vi "Message Parser Main.vi"(8 "error in (no error)":errorcluster, 11 "Message":T1={"Payload Size"=0, "Sequence Number"=0, "Sensor Type"=enum."APP", "Message Types"=enum."SEND_LOG_FILE_SIZE", "Data"=[]}) -> (0 "error out":errorcluster)   [LabVIEW 2019]
uses:
  Typedefs/Message.ctl
  Typedefs/Sensor Types.ctl
  Typedefs/Message Types.ctl
  Comms/State Controller/Controls/Comms Loop States.ctl
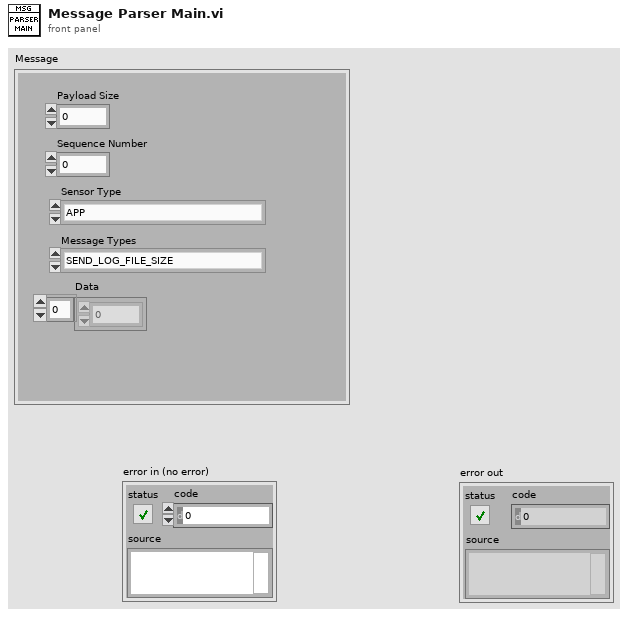
[diagram p1: front panel]
types:
  T1 = typedef "Message.ctl" = cluster{"Payload Size":u8, "Sequence Number":u8, "Sensor Type":T2, "Message Types":T3, "Data":u8[]}
  T2 = typedef "Sensor Types.ctl" = enum16{"APP", "TURBIDITY", "PH"}
  T3 = typedef "Message Types.ctl" = enum16{"HEART_BEAT", "CONNECT", "GET_CURRENT_MEASUREMENTS", "GET_LOG_FILE", "SEND_LOG_FILE_SIZE", "SEND_LOG_FILE_CHUNK", "GET_LOGGING_PERIOD", "SET_LOGGING_PERIOD", "SEND_SD_CARD_INFO", "GET_LOGS_LIST", "SEND_LOG_FILE_NAME", "SEND_LOGGING_PERIOD", "GET_RTC_TIME", "SET_RTC_TIME", "SEND_RTC_TIME", "SEND_CURRENT_MEASUREMENTS", "DELETE_LOG_FILE", "GET_SD_CARD_INFO", "GET_BATTERY_INFO", "SEND_BATTERY_INFO", "GET_LOG_FILE_SIZE", "SET_WIFI_SSID", "SET_WIFI_PASSWORD", "GET_WIFI_DETAILS", "SEND_WIFI_DETAILS", "ERROR_MSG"}
  T4 = typedef "Comms Loop States.ctl" = enum16{"Initalise", "User Event", "HEART_BEAT", "SEND_LOG_FILE_NAME", "Clear Log File Names", "SEND_LOG_FILE_CHUNK", "SEND_LOG_FILE_SIZE", "SEND_SD_CARD_INFO", "SEND_BATTERY_INFO", "SEND_LOGGING_PERIOD", "SEND_RTC_TIME", "SEND_CURRENT_MEASUREMENTS", "ERROR_MSG", "Clear Error Messages", "Send Message", "Idle", "Sensor Connected", "Sensor Disconnected", "Set Page Displayed", "Set Connected Sensor Type", "UI: Update Sensor Type", "UI: Update Log List", "Reset Log File Transfer", "SEND_WIFI_DETAILS"}
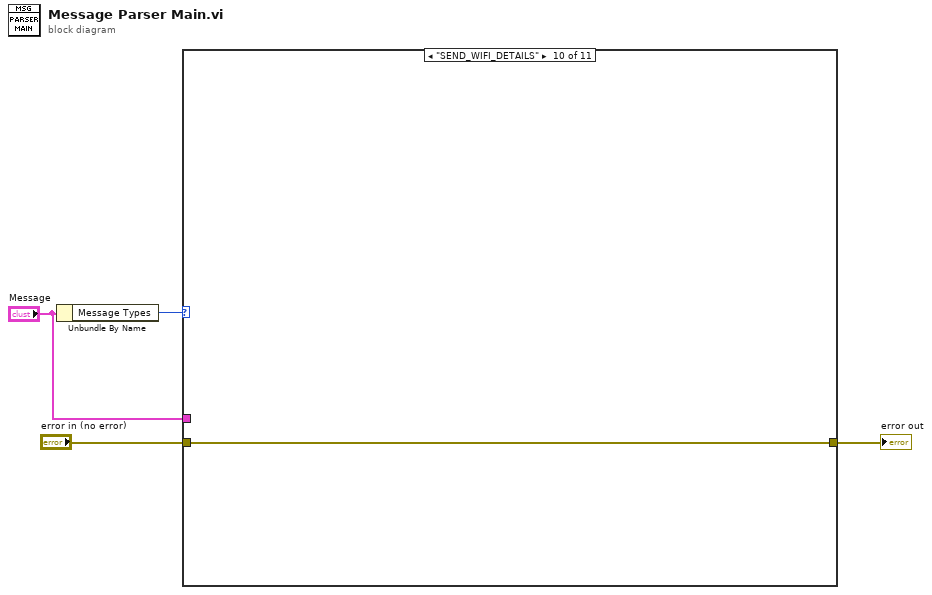
[diagram p0: block diagram]
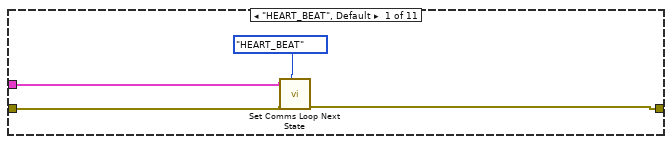
[diagram p2: hidden frame]
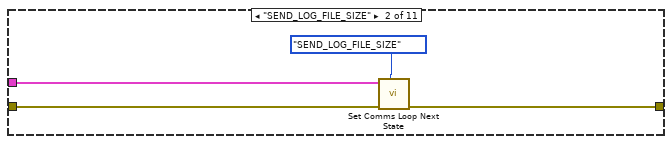
[diagram p3: hidden frame]
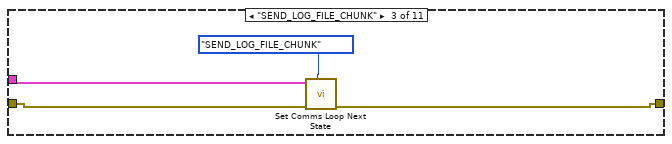
[diagram p4: hidden frame]
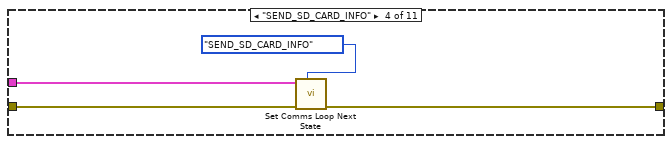
[diagram p5: hidden frame]
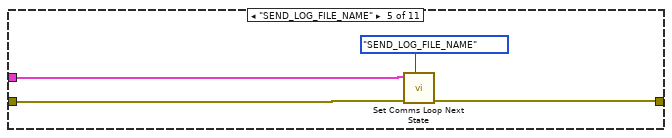
[diagram p6: hidden frame]
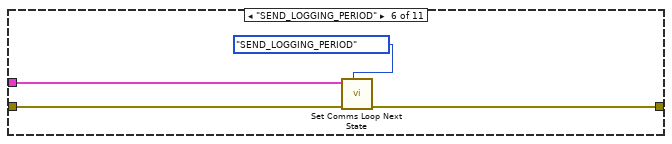
[diagram p7: hidden frame]
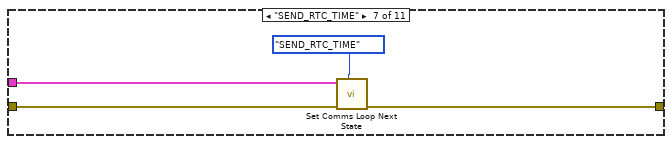
[diagram p8: hidden frame]
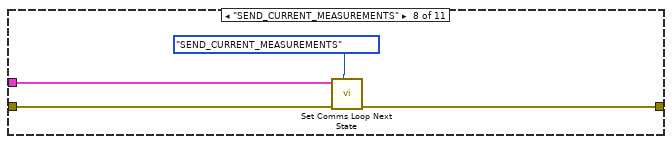
[diagram p9: hidden frame]
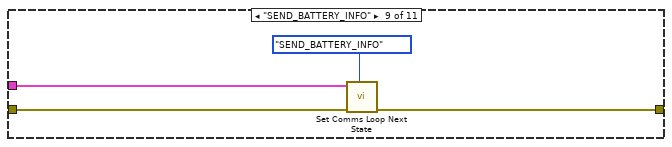
[diagram p10: hidden frame]
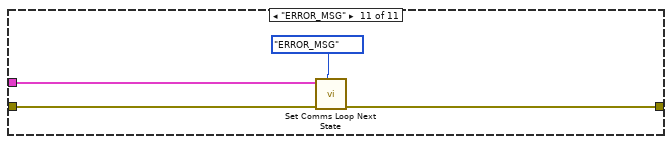
[diagram p11: hidden frame]
diagram:
  n1 = Unbundle By Name("Message") -> ("Message Types"=w2:T3)
  n2 = case shown="\"SEND_WIFI_DETAILS\"" w2 {
    tunnel: [w5 w9 w13 w17 w23 w25 w29 w34 w37 w41 w42] -> w4
    tunnel: "error in (no error)" -> [w7 w10 w15 w18 w22 w27 w31 w35 w39 w41 w44]
    tunnel: "Message" -> [w6 w11 w14 w19 w21 w26 w30 w33 w38 _ w43]
    frame "HEART_BEAT", Default {
      n3 = call "Set Comms Loop Next State.vi"("Command"=Comms_Loop_States."HEART_BEAT", "error in (no error)"=w7, "Data"=w6) -> ("error out"=w5:errorcluster)  [unwired: 8 in]
    }
    frame "SEND_LOG_FILE_SIZE" {
      n4 = call "Set Comms Loop Next State.vi"("Command"=Comms_Loop_States."SEND_LOG_FILE_SIZE", "error in (no error)"=w10, "Data"=w11) -> ("error out"=w9:errorcluster)  [unwired: 8 in]
    }
    frame "SEND_LOG_FILE_CHUNK" {
      n5 = call "Set Comms Loop Next State.vi"("Command"=Comms_Loop_States."SEND_LOG_FILE_CHUNK", "error in (no error)"=w15, "Data"=w14) -> ("error out"=w13:errorcluster)  [unwired: 8 in]
    }
    frame "SEND_SD_CARD_INFO" {
      n6 = call "Set Comms Loop Next State.vi"("Command"=Comms_Loop_States."SEND_SD_CARD_INFO", "error in (no error)"=w18, "Data"=w19) -> ("error out"=w17:errorcluster)  [unwired: 8 in]
    }
    frame "SEND_LOG_FILE_NAME" {
      n7 = call "Set Comms Loop Next State.vi"("Command"=Comms_Loop_States."SEND_LOG_FILE_NAME", "error in (no error)"=w22, "Data"=w21) -> ("error out"=w23:errorcluster)  [unwired: 8 in]
    }
    frame "SEND_LOGGING_PERIOD" {
      n8 = call "Set Comms Loop Next State.vi"("Command"=Comms_Loop_States."SEND_LOGGING_PERIOD", "error in (no error)"=w27, "Data"=w26) -> ("error out"=w25:errorcluster)  [unwired: 8 in]
    }
    frame "SEND_RTC_TIME" {
      n9 = call "Set Comms Loop Next State.vi"("Command"=Comms_Loop_States."SEND_RTC_TIME", "error in (no error)"=w31, "Data"=w30) -> ("error out"=w29:errorcluster)  [unwired: 8 in]
    }
    frame "SEND_CURRENT_MEASUREMENTS" {
      n10 = call "Set Comms Loop Next State.vi"("Command"=Comms_Loop_States."SEND_CURRENT_MEASUREMENTS", "error in (no error)"=w35, "Data"=w33) -> ("error out"=w34:errorcluster)  [unwired: 8 in]
    }
    frame "SEND_BATTERY_INFO" {
      n11 = call "Set Comms Loop Next State.vi"("Command"=Comms_Loop_States."SEND_BATTERY_INFO", "error in (no error)"=w39, "Data"=w38) -> ("error out"=w37:errorcluster)  [unwired: 8 in]
    }
    frame "SEND_WIFI_DETAILS" {
    }
    frame "ERROR_MSG" {
      n12 = call "Set Comms Loop Next State.vi"("Command"=Comms_Loop_States."ERROR_MSG", "error in (no error)"=w44, "Data"=w43) -> ("error out"=w42:errorcluster)  [unwired: 8 in]
    }
  }
  "error out" <- w4
